vi "Login.vi"(7 "Database":refnum<queue>, 8 "error in (no error)":errorcluster, 11 "System Config":T1 {"Config Settings"."Simulated Sensor Injection" scale=0.0..100.0}) -> (0 "error out":errorcluster, 3 "Simulation Mode?":bool)   [LabVIEW 2026, in "Admin.lvlib"]
uses:
  Admin/Admin.lvlib
  Architecture/Message Queue/Message Cluster.ctl
  controls/UI/System Config.ctl
  controls/UI/Config Settings.ctl
  controls/UI/Analog Output.ctl
  controls/UI/Units Enum.ctl
  controls/UI/Signal Enum.ctl
  controls/UI/Login Refs.ctl
  controls/UI/UI List Type.ctl
  controls/UI/Data Entity.ctl
  controls/Diagnostics/Error Payload.ctl
  controls/Diagnostics/Error Cluster.ctl
  controls/Messaging Payloads/Sensor InsertRequest.ctl
  controls/Messaging Payloads/Sensor CoreData Cluster.ctl
  controls/Messaging Payloads/Operator InsertRequest.ctl
  C:/Program Files (x86)/dotnet/shared/Microsoft.NETCore.App/8.0.22/System.Security.Cryptography.dll
  Program Files (x86)/dotnet/shared/Microsoft.NETCore.App/8.0.22/System.Security.Cryptography.dll
  Architecture/Message Queue/Enqueue Message (Single).vi
  Architecture/Message Queue/Message Queue.lvlib
  Settings/Settings.lvlib
panel:
  in  "Log Out":bool
  out "Message":string
  out "Status":bool
  in  "Tab Control":enum32{"Page 1", "Sensors", "Operators"}(tab)
  in  "OK Button":bool
  in  "Cancel Button":bool
  in  "Password":string
  in  "Output Signal":T4
  in  "Units":T5
  in  "Maximum":dbl
  in  "Minimum":dbl
  in  "Serial Number":string
  in  "Model Numbers":string(combo)
  in  "Submit":bool
  in  "Submit 2":bool
  in  "New Operator Name":string
  # "ADMINISTRATOR ACCESS"
  # "Enter you administrator password to continue."
  # "Administrator access is required to manage \n           sensors and operators."
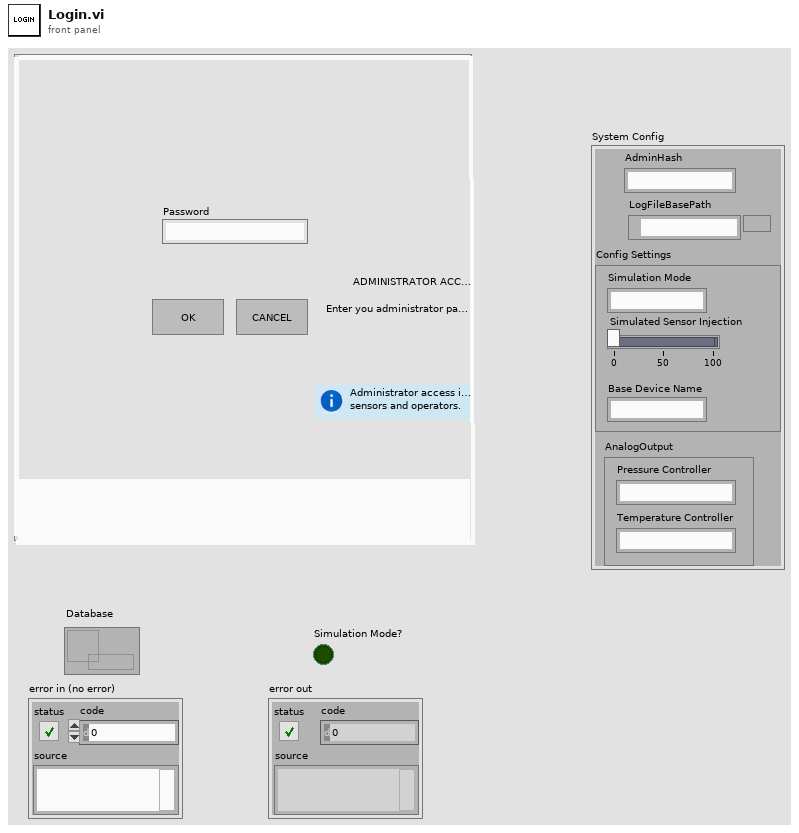
[diagram p1: front panel]
types:
  T1 = typedef "System Config.ctl" = cluster{"AdminHash":string, "LogFileBasePath ":path, "Config Settings":T2, "AnalogOutput":T3}
  T2 = typedef "Config Settings.ctl" = cluster{"Simulated Sensor Injection":dbl, "Base Device Name":string, "Simulation Mode":string}
  T3 = typedef "Settings.lvlib/Analog Output.ctl" = cluster{"Pressure Controller":string, "Temperature Controller":string}
  T4 = typedef "Signal Enum.ctl" = enum16{"4-20mA", "0-10V", "Thermocouple Type K"}
  T5 = typedef "Units Enum.ctl" = enum16{"PSI", "Deg C", "kPa", "GPM"}
  T6 = typedef "Login Refs.ctl" = cluster{"Serial Number Ref":refnum<vi>, "Submit Ref":refnum<vi>, "Clear Refnum ":refnum<vi>, "Logout Ref":refnum<vi>, "Message Ref":refnum<vi>, "Status Ref":refnum<vi>, "TabCtl Ref":refnum<vi>, "Submit Ref 2":refnum<vi>}
  T7 = typedef "Settings.lvlib/Data Entity.ctl" = enum16{"Measurement", "Controller", " Test Configuration"}
  T8 = enum8{"Enabled", "Disabled", "Disabled and Grayed Out"}
  T9 = typedef "UI List Type.ctl" = enum16{"Model Numbers", "Serial Numbers", "Operators", "Calibration Points", "Start Run Times"}
  T10 = typedef "Error Payload.ctl" = cluster{"Error Cluster":T11, "Message":string}
  T11 = typedef "Error Cluster.ctl" = errorcluster
  T12 = typedef "Sensor InsertRequest.ctl" = cluster{"Notifier":refnum<notifier>, "Sensor CoreData":T13}
  T13 = typedef "Settings.lvlib/Sensor CoreData Cluster.ctl" = cluster{"SerialNumber":string, "ModelNumber":string, "Min":dbl, "Max":dbl, "Units":T5, "Output Signal":T4, "SensorID":i32}
  T14 = typedef "Operator InsertRequest.ctl" = cluster{"Notifier":refnum<notifier>, "OperatorName":string, "BadgeNumber":string, "IsActive":i32}
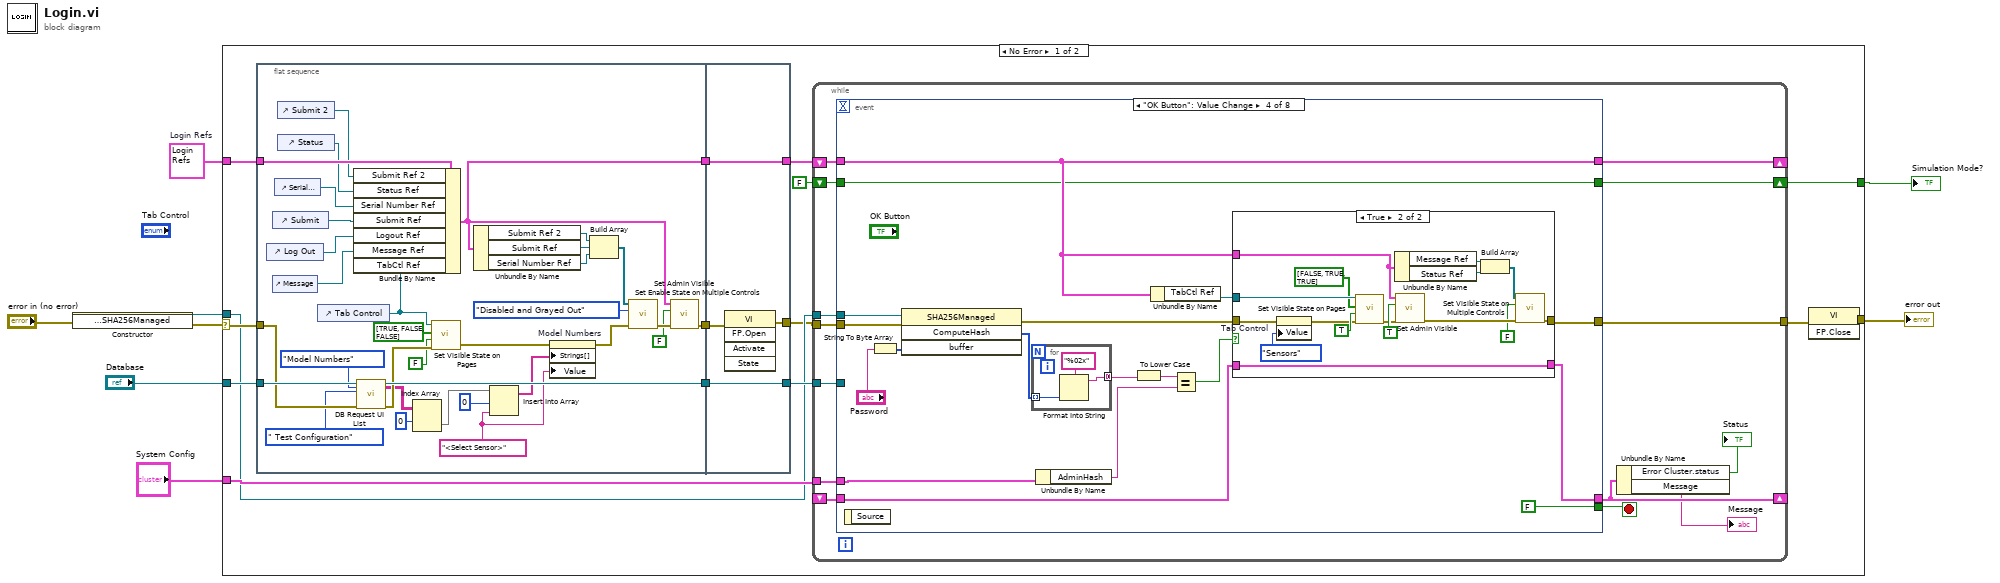
[diagram p0: block diagram]
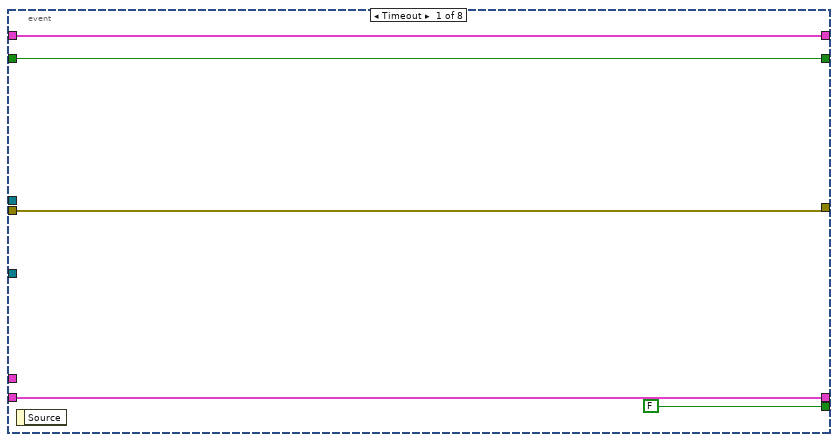
[diagram p2: hidden frame]
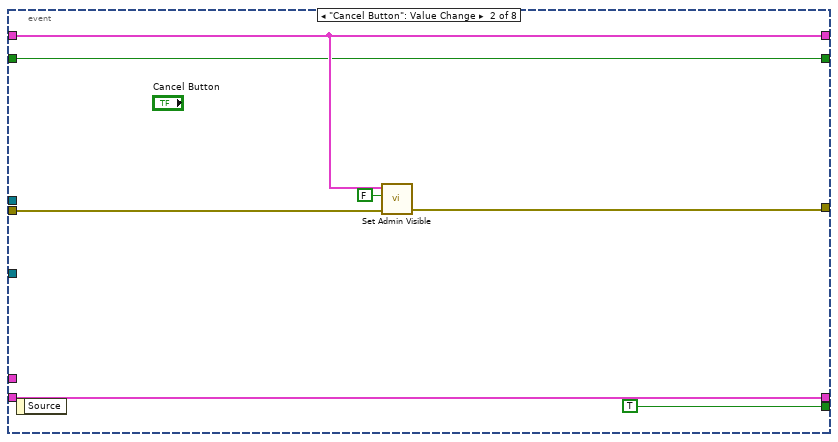
[diagram p3: hidden frame]
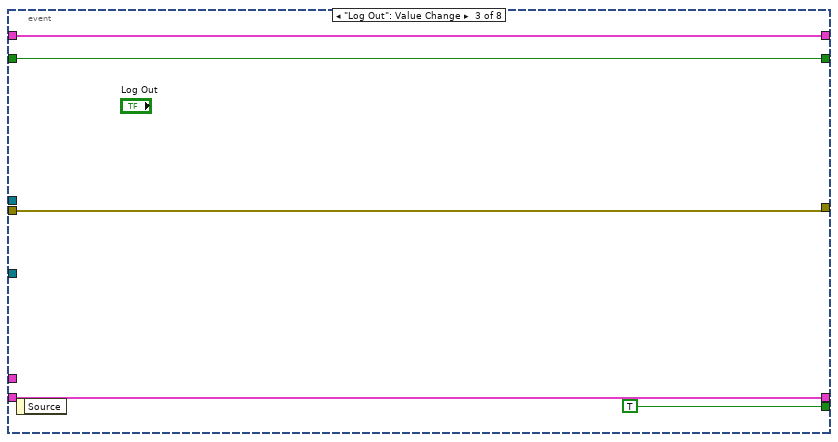
[diagram p4: hidden frame]
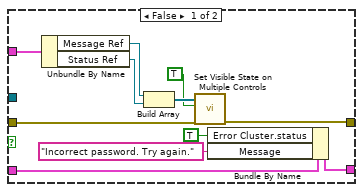
[diagram p5: hidden frame]
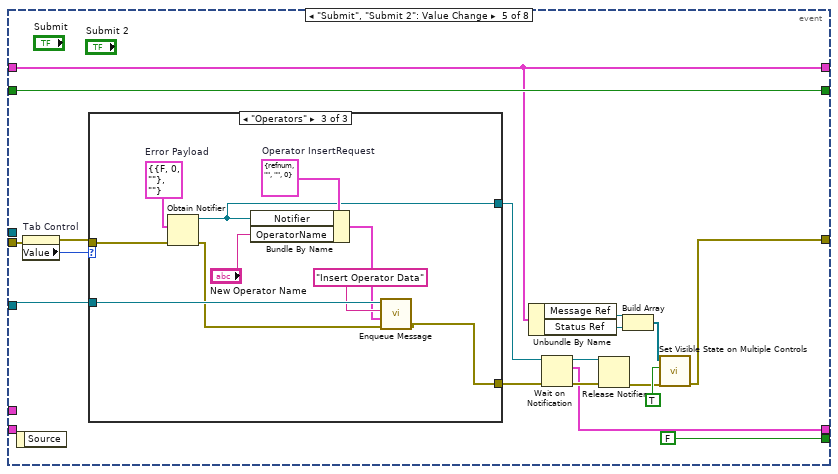
[diagram p6: hidden frame]
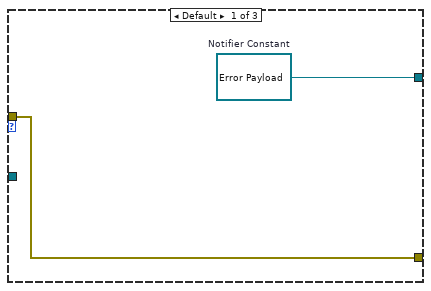
[diagram p7: hidden frame]
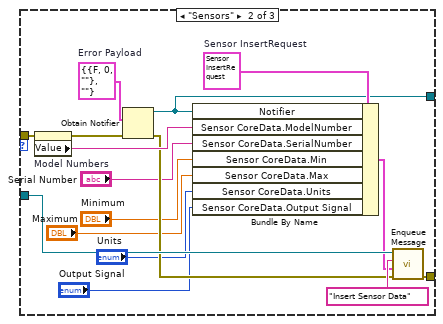
[diagram p8: hidden frame]
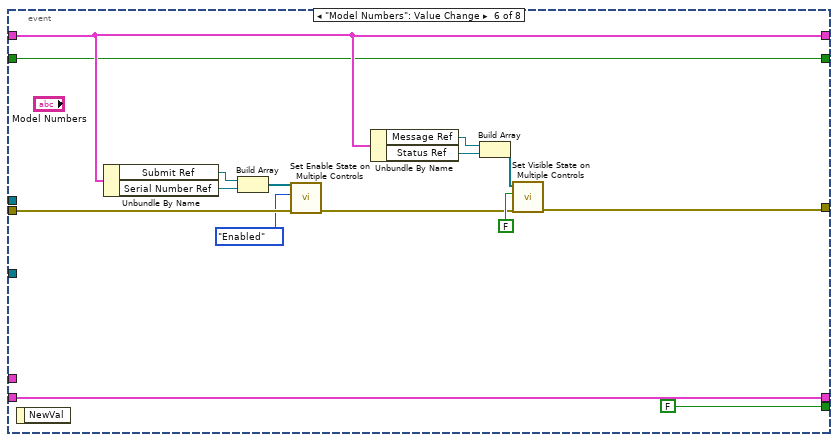
[diagram p9: hidden frame]
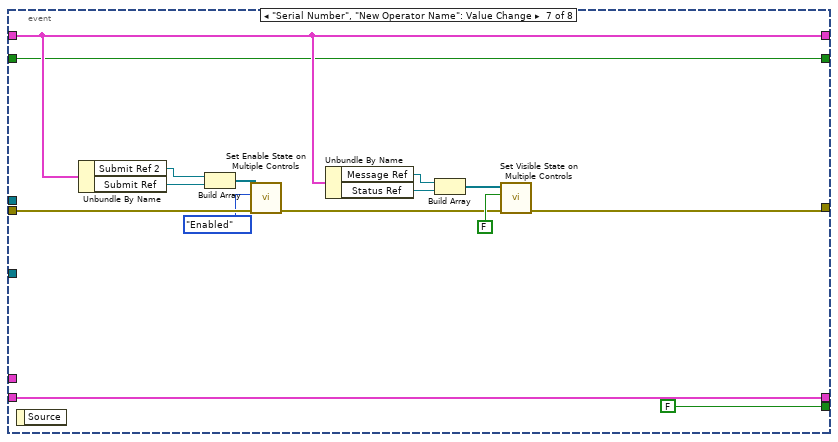
[diagram p10: hidden frame]
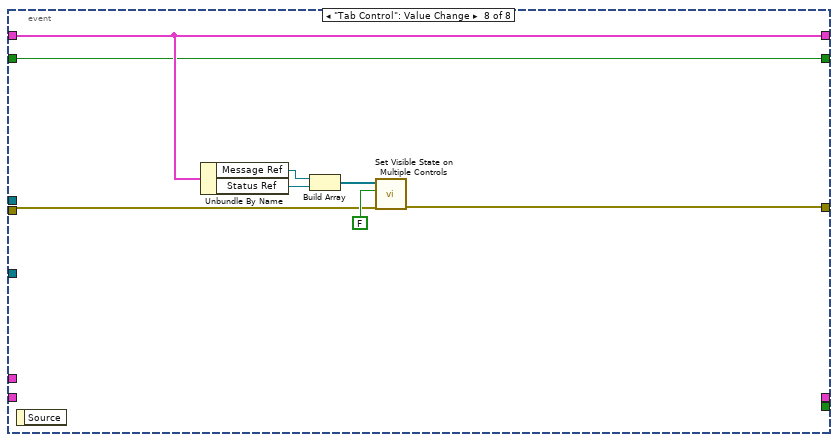
[diagram p11: hidden frame]
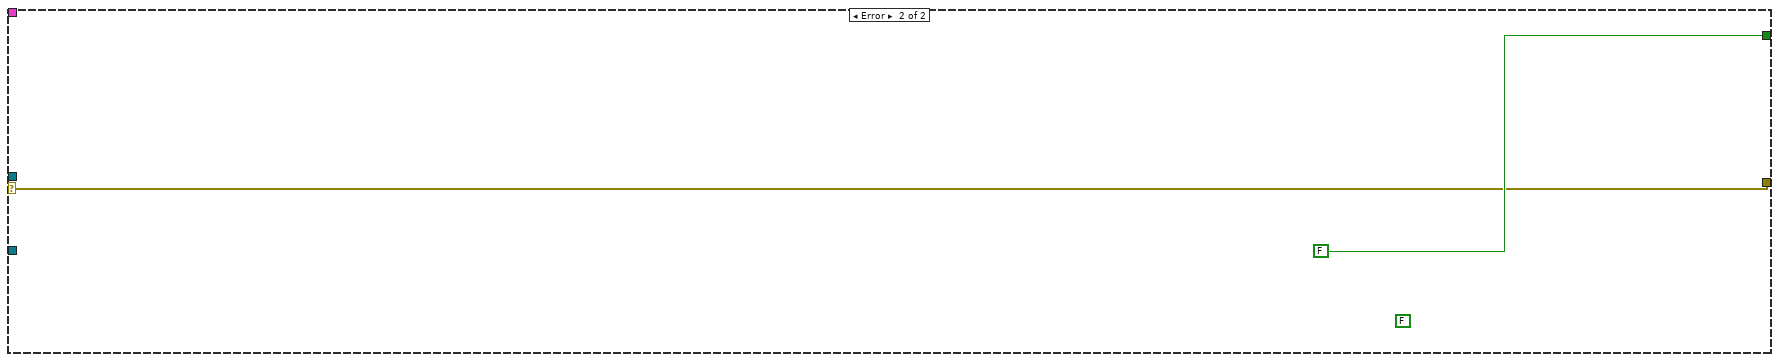
[diagram p12: hidden frame]
diagram:
  w3 = T6 {"Serial Number Ref"=refnum, "Submit Ref"=refnum, "Clear Refnum "=refnum, "Logout Ref"=refnum, "Message Ref"=refnum, "Status Ref"=refnum, "TabCtl Ref"=refnum, "Submit Ref 2"=refnum}  # Login Refs
  n1 = constructor class="SHA256Managed"(error in="error in (no error)") -> (reference out=w6:refnum<k39>, error out=w2:errorcluster)  [unwired: 2 in, 1 out]
  n2 = case shown="No Error" w2 {
    selector: w2 -> [w15 w224]
    tunnel: [w23 FALSE] -> w8
    tunnel: [w22 w224] -> w7
    tunnel: w6 -> [w14 _]
    tunnel: "Database" -> [w21 _]
    tunnel: w3 -> [w19 _]
    tunnel: "System Config" -> [w17 _]
    frame No Error {
      n3 = flat-sequence {
        tunnel: w21 -> [w56]
        tunnel: w19 -> [w51]
        tunnel: w15 -> [w33]
        tunnel: [w55] -> w13
        tunnel: [w40] -> w12
        tunnel: [w34] -> w11
        tunnel: [w59] -> w16
        tunnel: [w60] -> w20
        tunnel: w13 -> [w60]
        tunnel: w12 -> [w59]
        tunnel: w11 -> [w58]
        tunnel: [w57] -> w10
        frame #0 {
          w47 = "<Select Sensor>"
          n4 = control-ref of="Log Out"() -> (w52:refnum<vi>)
          n5 = control-ref of="Submit"() -> (w54:refnum<vi>)
          n6 = control-ref of="Message"() -> (w46:refnum<vi>)
          n7 = control-ref of="Serial Number"() -> (w53:refnum<vi>)
          n8 = control-ref of="Submit 2"() -> (w26:refnum<vi>)
          n9 = control-ref of="Status"() -> (w39:refnum<vi>)
          n10 = control-ref of="Tab Control"() -> (w27:refnum<vi>)
          n11 = Bundle By Name(cluster=w51, "Submit Ref 2"=w26, "Status Ref"=w39, "Serial Number Ref"=w53, "Submit Ref"=w54, "Logout Ref"=w52, "Message Ref"=w46, "TabCtl Ref"=w27) -> (w40:T6)
          n12 = call "DB Request UI List.vi"("Database in"=w56, "UI List Type"=UI_List_Type."Model Numbers", "UI Device Type"=Data_Entity." Test Configuration", "error in (no error)"=w33) -> ("Database out"=w55:refnum<queue>, "Results"=w29:string[][], "error out"=w38:errorcluster)  [unwired: 13 in]
          n13 = Index Array(array=w29, index (row)=0 ("index")) -> (element=w28:string[])  [unwired: 1 in]
          n14 = call "Set Visible State on Pages.vi"("error in (no error)"=w38, "Tabs Visible?"=FALSE, "Pages Visible"=bool[] [TRUE, FALSE, FALSE] ("Visibles"), "TabControl in"=w27) -> ("error out"=w37:errorcluster)  [unwired: 7 in]
          n15 = Unbundle By Name(w40) -> ("Submit Ref 2"=w25:refnum<vi>, "Submit Ref"=w43:refnum<vi>, "Serial Number Ref"=w42:refnum<vi>)
          n16 = Insert Into Array(array=w28, index=0, new element=w47) -> (w48:string[])
          n17 = property on="Model Numbers" class="CmbBox"(error in=w37, "Strings[]"=w48, "Value"=w47) -> (error out=w49:errorcluster)  [unwired: 1 in, 1 out]
          n18 = Build Array(w25, w43, w42) -> (w44:refnum<vi>[])
          n19 = call "Set Enable State on Multiple Controls.vi"("Controls"=w44, "Disabled"=T8."Disabled and Grayed Out", "error in (no error)"=w49) -> ("error out"=w45:errorcluster)  [unwired: 7 in]
          n20 = call "Set Admin Visible .vi"("error in (no error)"=w45, "Visible"=FALSE, "Login Refs"=w40) -> ("error out"=w34:errorcluster)  [unwired: 8 in]
        }
        frame #1 {
          n21 = invoke class="VI" method="FP.Open"(error in=w58) -> (error out=w57:errorcluster)  [unwired: 4 in, 4 out]
        }
      }
      n22 = while {
        tunnel: w17 -> [w73]
        tunnel: w14 -> [w72]
        tunnel: w20 -> [w71]
        tunnel: w10 -> [w70]
        shift-right: [w66] -> _
        shift-left: _ -> [w68]
        shift-right: [w63] -> _
        shift-left: w16 -> [w64]
        tunnel: [w62] -> w18
        shift-right: [w74] -> w23
        shift-left: FALSE ("Simulation Mode") -> [w61]
        stop <- w69 stop-if-true
        n23 = event shown="[3] \"OK Button\": Value Change" {
          selector: _ -> [_ _ _ _ _ _ _ _]
          dyn-events: _ -> [_ _ _ _ _ _ _ _]
          timeout: _ -> [_ _ _ _ _ _ _ _]
          tunnel: [w75 w80 w87 w96 w141 w188 w203 w216] -> w74
          tunnel: w73 -> [_ _ _ w103 _ _ _ _]
          tunnel: w72 -> [_ _ _ w108 _ _ _ _]
          tunnel: w70 -> [w78 w84 w90 w107 w149 w198 w213 w218]
          tunnel: w71 -> [_ _ _ _ w157 _ _ _]
          tunnel: [w78 w83 w90 w99 w143 w192 w204 w217] -> w62
          tunnel: [w77 w85 w89 w97 w151 w200 w215 _] -> w66
          tunnel: [FALSE ("status") TRUE TRUE FALSE FALSE ("status") FALSE ("status") FALSE ("status") _] -> w69
          tunnel: w68 -> [w77 w85 w89 w98 _ w200 w215 _]
          tunnel: w64 -> [w76 w82 w88 w100 w140 w191 w206 w219]
          tunnel: [w76 w82 w88 w100 w140 w191 w206 w219] -> w63
          tunnel: w61 -> [w75 w80 w87 w96 w141 w188 w203 w216]
          event Timeout {
            n24 = event-data() -> ()  [unwired: 1 in, 1 out]
          }
          event "Cancel Button": Value Change {
            n25 = event-data() -> ()  [unwired: 1 in, 1 out]
            n26 = call "Set Admin Visible .vi"("error in (no error)"=w84, "Visible"=FALSE, "Login Refs"=w82) -> ("error out"=w83:errorcluster)  [unwired: 8 in]
          }
          event "Log Out": Value Change {
            n27 = event-data() -> ()  [unwired: 1 in, 1 out]
          }
          event "OK Button": Value Change {
            n28 = event-data() -> ()  [unwired: 1 in, 1 out]
            n29 = String To Byte Array(string="Password") -> (unsigned byte array=w95:u8[])
            n30 = invoke class="SHA256Managed" method="ComputeHash"(reference=w108, error in=w107, "buffer"=w95) -> (error out=w105:errorcluster, "ComputeHash"=w94:u8[])  [unwired: 1 in, 2 out]
            n31 = for {
              tunnel: [w138] -> w93 mode=concatenating
              tunnel: w94 -> [w137] mode=indexing
              n32 = Format Into String(format string="%02x", w137) -> (resulting string=w138:string)  [unwired: 2 in, 1 out]
            }
            n33 = Unbundle By Name(w103) -> ("AdminHash"=w102:string)
            n34 = To Lower Case(string=w93) -> (all lower case string=w92:string)
            n35 = Unbundle By Name(w100) -> ("TabCtl Ref"=w101:refnum<vi>)
            n36 = Equal?(x=w92, y=w102) -> (x = y?=w106:bool)
            n37 = case shown="True" w106 {
              tunnel: w105 -> [w120 w123]
              tunnel: [w114 w125] -> w99
              tunnel: w101 -> [_ w136]
              tunnel: w100 -> [w119 w127]
              tunnel: w98 -> [w115 w124]
              tunnel: [w113 w124] -> w97
              frame False {
                n38 = Unbundle By Name(w119) -> ("Message Ref"=w118:refnum<vi>, "Status Ref"=w110:refnum<vi>)
                n39 = Build Array(w118, w110) -> (w117:refnum<vi>[])
                n40 = call "Set Visible State on Multiple Controls.vi"("error in (no error)"=w120, "Visible?"=TRUE, "Controls"=w117) -> ("error out"=w114:errorcluster)  [unwired: 8 in]
                n41 = Bundle By Name(cluster=w115, "Error Cluster.status"=TRUE, "Message"="Incorrect password. Try again.") -> (w113:T10)
              }
              frame True {
                n42 = property on="Tab Control" class="TabCtl (strict)"(error in=w123, "Value"=enum32{"Page 1", "Sensors", "Operators"}."Sensors" ("Tab Control")) -> (error out=w122:errorcluster)  [unwired: 1 in, 1 out]
                n43 = call "Set Visible State on Pages.vi"("error in (no error)"=w122, "Tabs Visible?"=TRUE, "Pages Visible"=bool[] [FALSE, TRUE, TRUE] ("Visibles"), "TabControl in"=w136) -> ("error out"=w126:errorcluster)  [unwired: 7 in]
                n44 = Unbundle By Name(w127) -> ("Message Ref"=w128:refnum<vi>, "Status Ref"=w131:refnum<vi>)
                n45 = call "Set Admin Visible .vi"("error in (no error)"=w126, "Visible"=TRUE, "Login Refs"=w127) -> ("error out"=w132:errorcluster)  [unwired: 8 in]
                n46 = Build Array(w128, w131) -> (w130:refnum<vi>[])
                n47 = call "Set Visible State on Multiple Controls.vi"("error in (no error)"=w132, "Visible?"=FALSE, "Controls"=w130) -> ("error out"=w125:errorcluster)  [unwired: 8 in]
              }
            }
          }
          event "Submit", "Submit 2": Value Change {
            n48 = event-data() -> ()  [unwired: 1 in, 1 out]
            n49 = property on="Tab Control" class="TabCtl (strict)"(error in=w149) -> (error out=w148:errorcluster, "Value"=w150:enum32{"Page 1", "Sensors", "Operators"})  [unwired: 1 in, 1 out]
            n50 = case shown="\"Operators\"" w150 {
              tunnel: w157 -> [_ w175 w185]
              tunnel: w148 -> [w159 w171 w177]
              tunnel: [w159 w169 w176] -> w155
              tunnel: [w158 w162 w179] -> w153
              frame Default {
                w158 = refnum<notifier> refnum  # Notifier Constant
              }
              frame "Sensors" {
                w166 = T10 {"Error Cluster"={"status"=FALSE, "code"=0, "source"=""}, "Message"=""}  # Error Payload
                w173 = T12 {"Notifier"=refnum, "Sensor CoreData"={"SerialNumber"="", "ModelNumber"="", "Min"=0.0, "Max"=0.0, "Units"=enum."PSI", "Output Signal"=enum."4-20mA", "SensorID"=0}}  # Sensor InsertRequest
                n51 = property on="Model Numbers" class="CmbBox"(error in=w171) -> (error out=w170:errorcluster, "Value"=w168:string)  [unwired: 1 in, 1 out]
                n52 = Obtain Notifier(notification data type=w166, error in (no error)=w170) -> (notifier out=w162:refnum<notifier>, error out=w167:errorcluster)  [unwired: 2 in, 1 out]
                n53 = Bundle By Name(cluster=w173, "Notifier"=w162, "Sensor CoreData.ModelNumber"=w168, "Sensor CoreData.SerialNumber"="Serial Number", "Sensor CoreData.Min"="Minimum", "Sensor CoreData.Max"="Maximum", "Sensor CoreData.Units"="Units", "Sensor CoreData.Output Signal"="Output Signal") -> (w172:T12)
                n54 = call-poly "Enqueue Message.vi"("error in (no error)"=w167, "Message Data"=w172, "Message"="Insert Sensor Data", "Message Queue"=w175) -> ("error out"=w169:errorcluster)  [unwired: 6 in, 1 out]
              }
              frame "Operators" {
                w180 = T10 {"Error Cluster"={"status"=FALSE, "code"=0, "source"=""}, "Message"=""}  # Error Payload
                w183 = T14 {"Notifier"=refnum, "OperatorName"="", "BadgeNumber"="", "IsActive"=0}  # Operator InsertRequest
                n55 = Obtain Notifier(notification data type=w180, error in (no error)=w177) -> (notifier out=w179:refnum<notifier>, error out=w181:errorcluster)  [unwired: 2 in, 1 out]
                n56 = Bundle By Name(cluster=w183, "Notifier"=w179, "OperatorName"="New Operator Name") -> (w182:T14)
                n57 = call-poly "Enqueue Message.vi"("error in (no error)"=w181, "Message Data"=w182, "Message"="Insert Operator Data", "Message Queue"=w185) -> ("error out"=w176:errorcluster)  [unwired: 6 in, 1 out]
              }
            }
            n58 = Unbundle By Name(w140) -> ("Message Ref"=w142:refnum<vi>, "Status Ref"=w147:refnum<vi>)
            n59 = Wait on Notification(notifier=w153, error in (no error)=w155) -> (notifier out=w154:refnum<notifier>, notification=w151:T10, error out=w156:errorcluster)  [unwired: 2 in, 1 out]
            n60 = Release Notifier(notifier=w154, error in (no error)=w156) -> (error out=w144:errorcluster)  [unwired: 1 in, 2 out]
            n61 = Build Array(w142, w147) -> (w146:refnum<vi>[])
            n62 = call "Set Visible State on Multiple Controls.vi"("error in (no error)"=w144, "Visible?"=TRUE, "Controls"=w146) -> ("error out"=w143:errorcluster)  [unwired: 8 in]
          }
          event "Model Numbers": Value Change {
            n63 = event-data() -> ()  [unwired: 1 in, 1 out]
            n64 = Unbundle By Name(w191) -> ("Submit Ref"=w187:refnum<vi>, "Serial Number Ref"=w197:refnum<vi>)
            n65 = Build Array(w187, w197) -> (w196:refnum<vi>[])
            n66 = call "Set Enable State on Multiple Controls.vi"("Controls"=w196, "Disabled"=T8."Enabled", "error in (no error)"=w198) -> ("error out"=w193:errorcluster)  [unwired: 7 in]
            n67 = Unbundle By Name(w191) -> ("Message Ref"=w189:refnum<vi>, "Status Ref"=w190:refnum<vi>)
            n68 = Build Array(w189, w190) -> (w195:refnum<vi>[])
            n69 = call "Set Visible State on Multiple Controls.vi"("error in (no error)"=w193, "Visible?"=FALSE, "Controls"=w195) -> ("error out"=w192:errorcluster)  [unwired: 8 in]
          }
          event "Serial Number", "New Operator Name": Value Change {
            n70 = event-data() -> ()  [unwired: 1 in, 1 out]
            n71 = Unbundle By Name(w206) -> ("Submit Ref 2"=w201:refnum<vi>, "Submit Ref"=w211:refnum<vi>)
            n72 = Build Array(w201, w211) -> (w212:refnum<vi>[])
            n73 = call "Set Enable State on Multiple Controls.vi"("Controls"=w212, "Disabled"=T8."Enabled", "error in (no error)"=w213) -> ("error out"=w205:errorcluster)  [unwired: 7 in]
            n74 = Unbundle By Name(w206) -> ("Message Ref"=w207:refnum<vi>, "Status Ref"=w208:refnum<vi>)
            n75 = Build Array(w207, w208) -> (w210:refnum<vi>[])
            n76 = call "Set Visible State on Multiple Controls.vi"("error in (no error)"=w205, "Visible?"=FALSE, "Controls"=w210) -> ("error out"=w204:errorcluster)  [unwired: 8 in]
          }
          event "Tab Control": Value Change {
            n77 = event-data() -> ()  [unwired: 1 in, 1 out]
            n78 = Unbundle By Name(w219) -> ("Message Ref"=w220:refnum<vi>, "Status Ref"=w221:refnum<vi>)
            n79 = Build Array(w220, w221) -> (w223:refnum<vi>[])
            n80 = call "Set Visible State on Multiple Controls.vi"("error in (no error)"=w218, "Visible?"=FALSE, "Controls"=w223) -> ("error out"=w217:errorcluster)  [unwired: 8 in]
          }
        }
        n81 = Unbundle By Name(w66) -> ("Error Cluster.status"=→"Status":bool, "Message"=→"Message":string)
      }
      n82 = invoke class="VI" method="FP.Close"(error in=w18) -> (error out=w22:errorcluster)  [unwired: 2 in, 2 out]
    }
    frame Error {
      (unwired) FALSE ("status")
    }
  }
  "error out" <- w7
  "Simulation Mode?" <- w8
